vi "CTU_ext.vi"(4 "DO old":u32, 5 "R":bool, 6 "DI":u32, 7 "IN":bool) -> (1 "DO":u32, 2 "EU":bool)   [LabVIEW 2019, in "Counter.lvlib"]
uses:
  Counter.lvlib
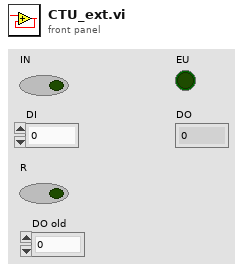
[diagram p1: front panel]
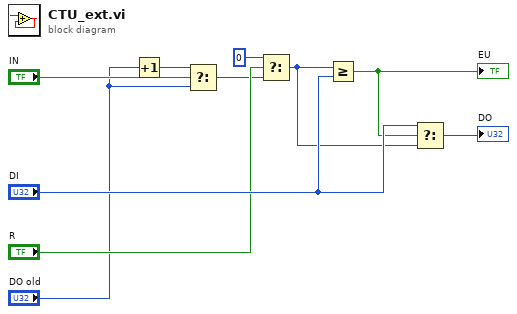
[diagram p0: block diagram]
diagram:
  n1 = Increment(x="DO old") -> (x+1=w3:u32)
  n2 = Select(t=w3, s="IN", f="DO old") -> (s? t:f=w2:u32)
  n3 = Select(t=u32 0, s="R", f=w2) -> (s? t:f=w5:u32)
  n4 = Greater Or Equal?(x=w5, y="DI") -> (x >= y?=w9:bool)
  "EU" <- w9
  n5 = Select(t="DI", s=w9, f=w5) -> (s? t:f=→"DO":u32)
